vi "subtract.vi"(8 "error in (no error)":errorcluster, 10 "subtrahend":refnum<class "Image.lvclass">, 11 "Image in":refnum<class "Image.lvclass">) -> (0 "error out":errorcluster, 3 "Image out":refnum<class "Image.lvclass">)   [LabVIEW 2010, in "Image.lvclass"]
uses:
  Image.lvclass
  storage_mode.ctl
  ErrorController/ErrorController/class_data.vi
  <vilib>/vision/NI_Vision_Development_Module.lvlib
  ErrorController/ErrorController/ErrorController.lvclass
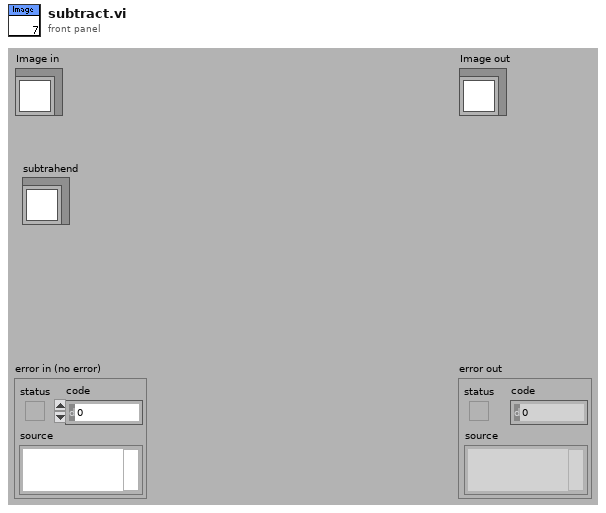
[diagram p1: front panel]
types:
  T1 = typedef "Image.lvclass/storage_mode.ctl" = enum16{"RAM", "disk"}
  T2 = typedef "IMAQ Image.ctl" = refnum<image>
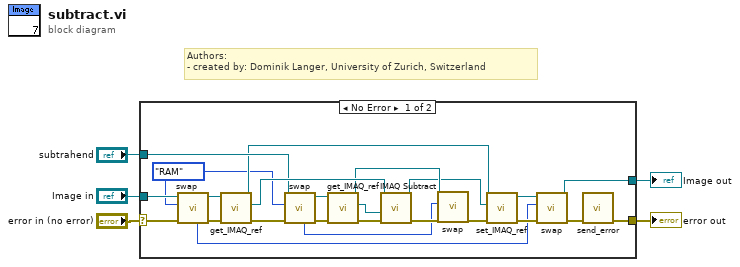
[diagram p0: block diagram]
diagram:
  # "Authors: \n- created by: Dominik Langer, University of Zurich, Switzerland"
  n1 = case shown="No Error" "error in (no error)" {
    selector: "error in (no error)" -> [w26 w31]
    tunnel: [w6 w31] -> w4
    tunnel: [w18 w30] -> w2
    tunnel: "Image in" -> [w29 w30]
    tunnel: "subtrahend" -> [w20 _]
    frame No Error {
      w9 = storage_mode."RAM" ("storage type target")
      n2 = call-dynamic "swap.vi"("error in (no error)"=w26, "storage type target"=w9, "Image in"=w29) -> ("error out"=w27:errorcluster, "Image out"=w28:refnum<class "Image.lvclass">, "previous storage mode"=w11:T1)  [unwired: 6 out]
      n3 = call-dynamic "get_IMAQ_ref.vi"("error in (no error)"=w27, "Image.lvclass in"=w28) -> ("error out"=w22:errorcluster, "Image"=w25:T2, "Image.lvclass out"=w17:refnum<class "Image.lvclass">)  [unwired: 7 out]
      n4 = call-dynamic "swap.vi"("error in (no error)"=w22, "storage type target"=w9, "Image in"=w20) -> ("error out"=w23:errorcluster, "Image out"=w24:refnum<class "Image.lvclass">, "previous storage mode"=w13:T1)  [unwired: 6 out]
      n5 = call-dynamic "get_IMAQ_ref.vi"("error in (no error)"=w23, "Image.lvclass in"=w24) -> ("error out"=w21:errorcluster, "Image"=w8:T2, "Image.lvclass out"=w12:refnum<class "Image.lvclass">)  [unwired: 7 out]
      n6 = call "IMAQ Subtract"("Image Src A"=w25, "Image Src B"=w8, "error in (no error)"=w21) -> ("Image Dst Out"=w10:T2, "error out"=w15:errorcluster)  [unwired: 2 in, 2 out]
      n7 = call-dynamic "swap.vi"("error in (no error)"=w15, "storage type target"=w13, "Image in"=w12) -> ("error out"=w14:errorcluster)  [unwired: 8 out]
      n8 = call-dynamic "set_IMAQ_ref.vi"("error in (no error)"=w14, "Image"=w10, "Image.lvclass in"=w17) -> ("error out"=w16:errorcluster, "Image.lvclass out"=w19:refnum<class "Image.lvclass">)  [unwired: 7 out]
      n9 = call-dynamic "swap.vi"("error in (no error)"=w16, "storage type target"=w11, "Image in"=w19) -> ("error out"=w7:errorcluster, "Image out"=w18:refnum<class "Image.lvclass">)  [unwired: 7 out]
      n10 = call "send_error.vi"("error in (no error)"=w7) -> ("error out"=w6:errorcluster)  [unwired: 10 in]
    }
    frame Error {
    }
  }
  "error out" <- w4
  "Image out" <- w2
